vi "testLoad.vi"() -> ()   [LabVIEW 2025]
uses:
  <vilib>/userDefined/High Color/IMAQdx.ctl
  <vilib>/vision/driver/NI_Vision_Acquisition_Software.lvlib
panel:
  out "Pixel Pointer out":u64 format="%.0x"
  out "After Img 2":T1(plugin-control)
  out "Refnum out 2":T2
  out "Refnum out":T2
  out "Width":u32
  out "Height":u32
  in  "Resolution Selection 2":u16(ring)=10 items=["640x480 MJPG 30.00fps", "1280x720 MJPG 30.00fps", "1920x1080 MJPG 30.00fps", "1920x1088 MJPG 30.00fps"]
  out "video Mode names 2":string[](array[string])
  in  "Camera Selection 2":string(combo)="cam5"
  out "Camera Index list 2":string[](array[string])
  out "loadedModel":string
  out "opencvCUDA":string
  out "HostDevice":string
  in  "Sensitivity adpThScl":sgl=1.5
  out "After Img":T1(plugin-control)
  in  "stop":bool
  in  "OK Button":bool
  in  "Resolution Selection":u16(ring)=10 items=["640x480 MJPG 30.00fps", "640x480 YUY2 30.00fps", "1280x720 MJPG 30.00fps", "1280x720 YUY2 7.50fps", "1920x1080 MJPG 30.00fps", "1920x1080 YUY2 2.00fps", "2048x1536 MJPG 30.00fps", "2048x1536 YUY2 2.00fps", "2560x1440 MJPG 30.00fps", "2560x1440 YUY2 2.00fps", "3840x2160 MJPG 30.00fps", "3840x2160 YUY2 1.00fps"]
  out "video Mode names":string[](array[string])
  in  "Camera Selection":string(combo)="cam5"
  in  "confirm camera":bool
  out "Camera Index list":string[](array[string])
  out "calAdpMsg":string
  in  "Cal Img Folder Path":path=path "D:/labviewTestTCVdll/AnomalyDetection-LabVIEW/testFolder"
  out "mBBMesg":string
  out "success 2":i32
  out "successFea":u32
  out "bufferMsg":string
  out "buffer":string
  out "appended path":path
  in  "modelPath":path=path "D:/labviewTestTCVdll/AnomalyDetection-LabVIEW/models/resnet50_fp32.ts"
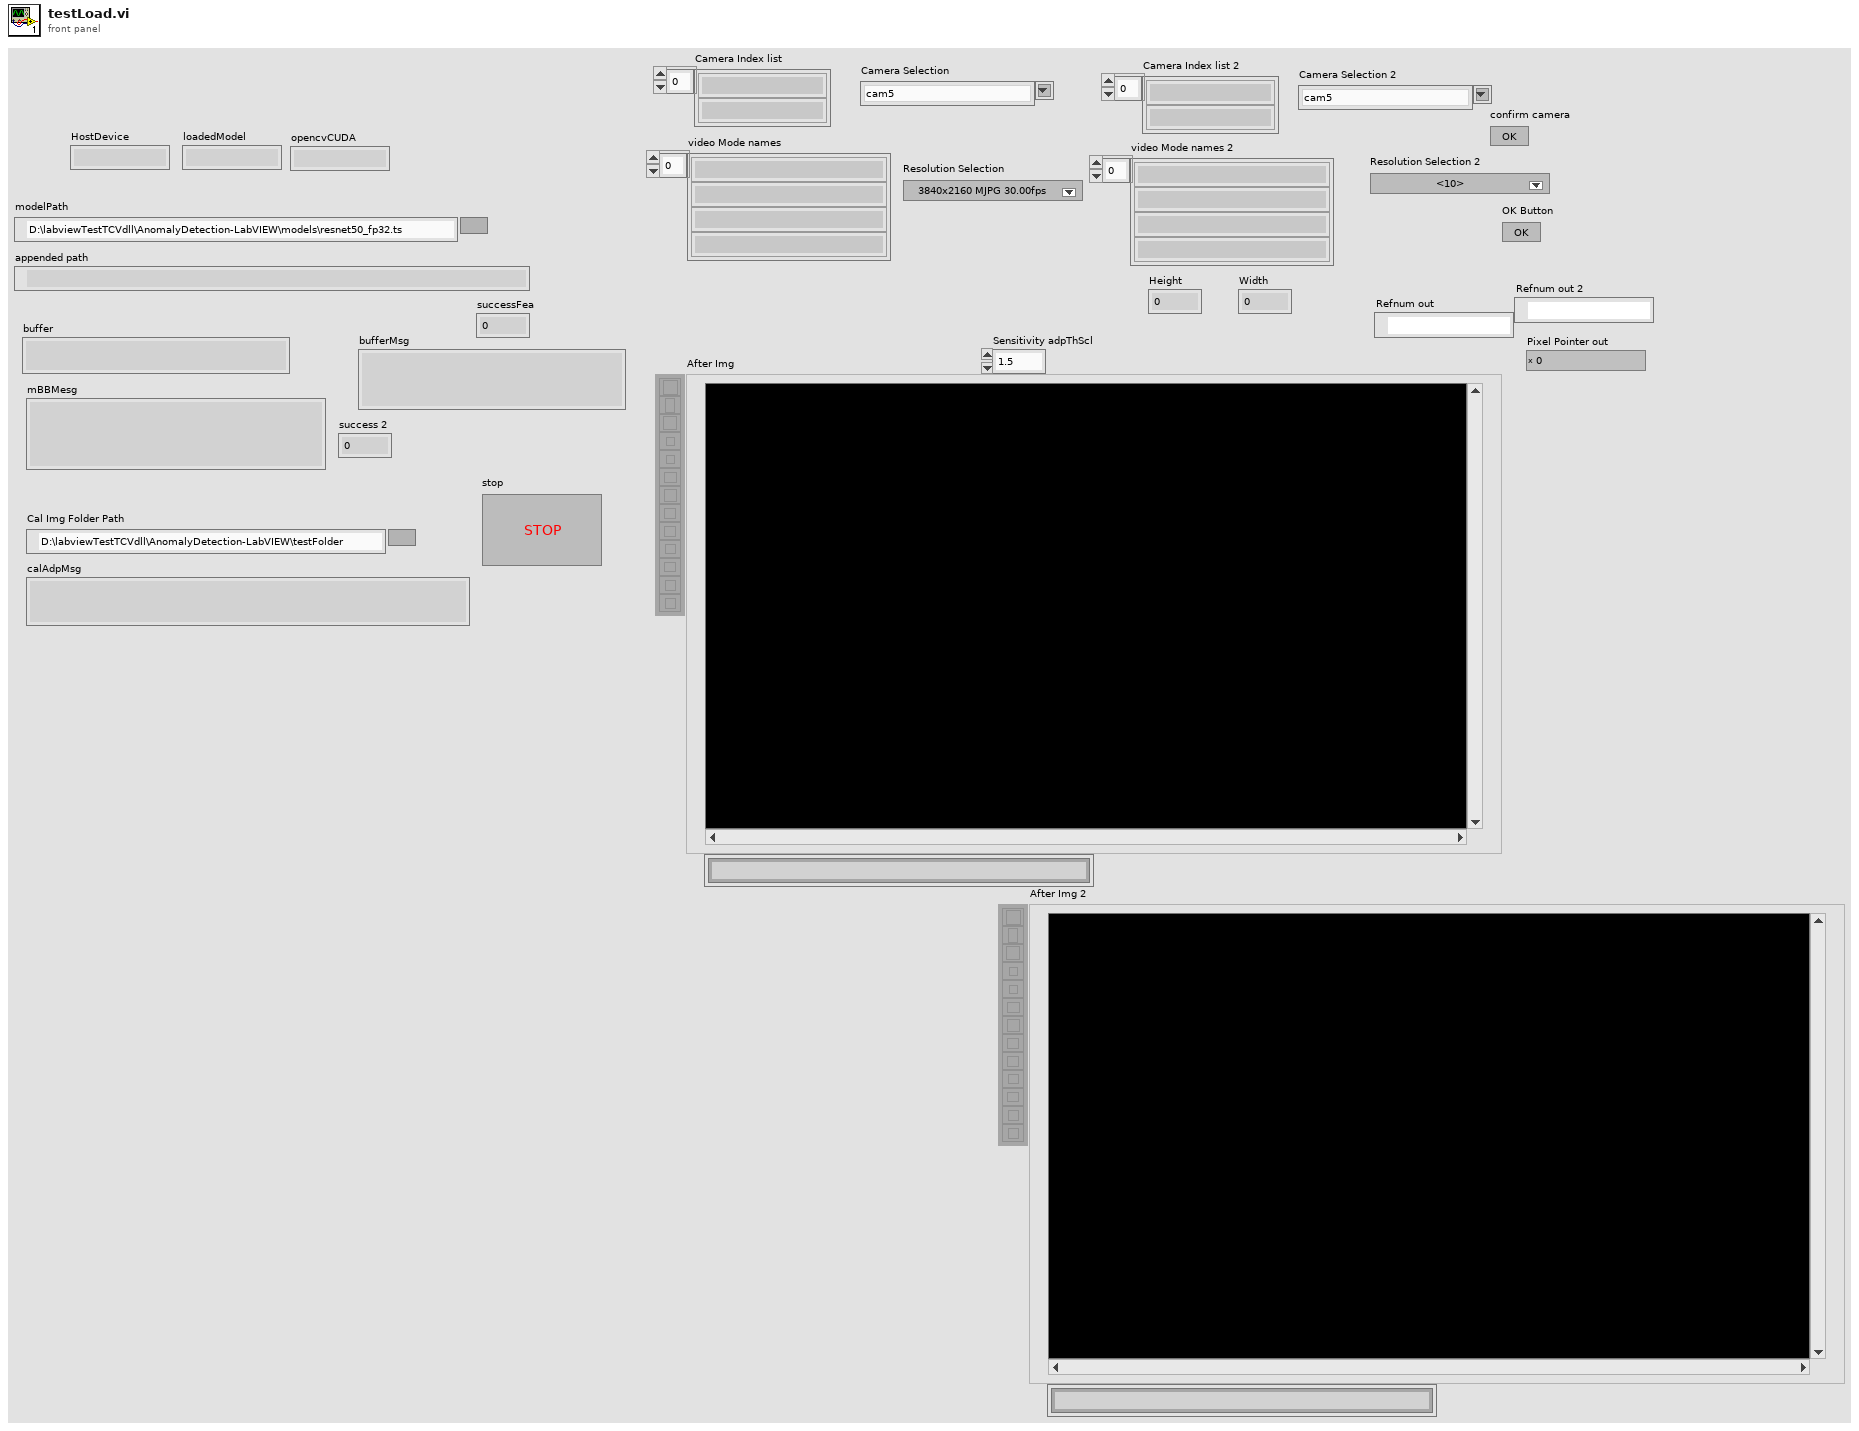
[diagram p1: front panel]
types:
  T1 = typedef "IMAQ Image.ctl" = refnum<image>
  T2 = typedef "IMAQdx.ctl" = refnum<k21>
  T3 = cluster{"Video Mode":u32, "Video Mode Name":string}[]
  T4 = enum32{"Map Pixel Pointer", "Unmap Pixel Pointer", "Get Pixels Infos"}
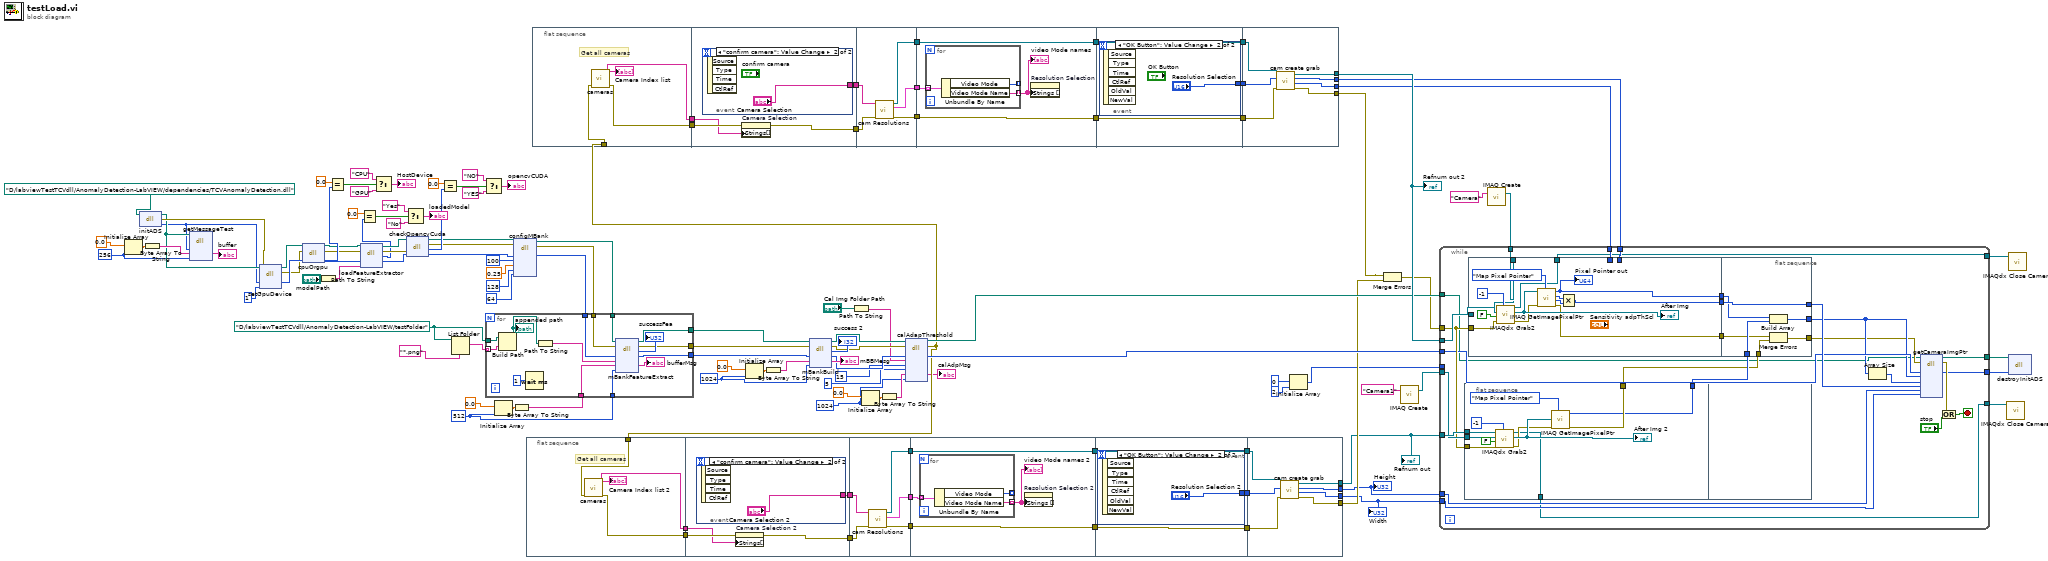
[diagram p0: block diagram]
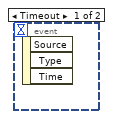
[diagram p2: hidden frame]
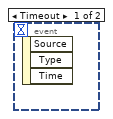
[diagram p3: hidden frame]
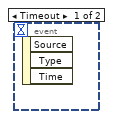
[diagram p4: hidden frame]
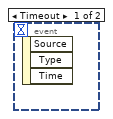
[diagram p5: hidden frame]
diagram:
  w20 = 1024 ("dimension size")
  w27 = 1024 ("dimension size")
  w33 = 512 ("dimension size")
  w5 = path "D:/labviewTestTCVdll/AnomalyDetection-LabVIEW/testFolder"
  w80 = 256 ("dimension size")
  n1 = Initialize Array(0.0 ("element"), w80) -> (w84:dbl[])
  n2 = dll-call lib="D:/labviewTestTCVdll/AnomalyDetection-LabVIEW/dependencies/TCVAnomalyDetection.dll" fn="initADS"(path in=path "D:/labviewTestTCVdll/AnomalyDetection-LabVIEW/dependencies/TCVAnomalyDetection.dll") -> (path out=w82:path, error out=w85:errorcluster, "ref"=w81:u64)  [unwired: 2 in]
  n3 = Byte Array To String(unsigned byte array=w84) -> (string=w83:string)
  n4 = dll-call lib="D:/labviewTestTCVdll/AnomalyDetection-LabVIEW/dependencies/TCVAnomalyDetection.dll" fn="getMessageTest"(path in=w82, "ref"=w81, "buffer"=w83, "size"=w80) -> ("buffer"=→"buffer":string)  [unwired: 5 in, 2 out]
  n5 = dll-call lib="D:/labviewTestTCVdll/AnomalyDetection-LabVIEW/dependencies/TCVAnomalyDetection.dll" fn="setGpuDevice"(path in=w82, error in=w85, "ref"=w81, "num"=u32 1) -> (path out=w57:path, error out=w56:errorcluster, "ref"=w58:u64)  [unwired: 3 in]
  n6 = dll-call lib="D:/labviewTestTCVdll/AnomalyDetection-LabVIEW/dependencies/TCVAnomalyDetection.dll" fn="cpuOrgpu"(path in=w57, error in=w56, "ref"=w58) -> (path out=w55:path, error out=w54:errorcluster, "ref"=w76:u64)  [unwired: 2 in]
  n7 = Path To String(path="modelPath") -> (string=w52:string)
  n8 = Equal?(x=0.0, y=w76) -> (x = y?=w75:bool)
  n9 = dll-call lib="D:/labviewTestTCVdll/AnomalyDetection-LabVIEW/dependencies/TCVAnomalyDetection.dll" fn="loadFeatureExtractor"(path in=w55, error in=w54, "ref"=w76, "path"=w52) -> (path out=w51:path, error out=w47:errorcluster, "success"=w6:i32, "ref"=w50:u64)  [unwired: 2 in]
  n10 = Equal?(x=0.0, y=w6) -> (x = y?=w8:bool)
  n11 = Select(t="CPU", s=w75, f="GPU") -> (s? t:f=→"HostDevice":string)
  n12 = dll-call lib="D:/labviewTestTCVdll/AnomalyDetection-LabVIEW/dependencies/TCVAnomalyDetection.dll" fn="checkOpencvCuda"(path in=w51, error in=w47, "ref"=w50) -> (path out=w45:path, error out=w46:errorcluster, "ocvC"=w66:i32, "ref"=w44:u64)  [unwired: 1 in]
  n13 = Select(t="Yes", s=w8, f="No") -> (s? t:f=→"loadedModel":string)
  n14 = Equal?(x=0.0, y=w66) -> (x = y?=w68:bool)
  n15 = List Folder(path=w5, pattern="*.png") -> (filenames=w48:string[])  [unwired: 2 in, 3 out]
  n16 = Select(t="NO", s=w68, f="YES") -> (s? t:f=→"opencvCUDA":string)
  n17 = Initialize Array(0.0 ("element"), w33) -> (w39:dbl[])
  n18 = Byte Array To String(unsigned byte array=w39) -> (string=w34:string)
  n19 = dll-call lib="D:/labviewTestTCVdll/AnomalyDetection-LabVIEW/dependencies/TCVAnomalyDetection.dll" fn="configMBank"(path in=w45, error in=w46, "ref"=w44, "noImages"=u32 100, "coreset"=sgl 0.25, "patchSize"=u32 128, "pathStride"=u32 64) -> (path out=w37:path, error out=w36:errorcluster, "ref"=w35:u64)  [unwired: 6 in]
  n20 = for {
    tunnel: w5 -> [w138]
    tunnel: w48 -> [w137] mode=indexing
    tunnel: w37 -> [w136]
    tunnel: w36 -> [w135]
    tunnel: w35 -> [w134]
    tunnel: w34 -> [w131]
    tunnel: w33 -> [w130]
    tunnel: [w127] -> w30
    tunnel: [w126] -> w29
    tunnel: [w125] -> w24
    n21 = Build Path(base path=w138, name or relative path=w137) -> (appended path=w133:path)
    "appended path" <- w133
    n22 = Wait (ms)(milliseconds to wait=u32 1) -> ()  [unwired: 1 out]
    n23 = Path To String(path=w133) -> (string=w132:string)
    n24 = dll-call lib="D:/labviewTestTCVdll/AnomalyDetection-LabVIEW/dependencies/TCVAnomalyDetection.dll" fn="mBankFeatureExtract"(path in=w136, error in=w135, "ref"=w134, "imagePath"=w132, "bufferMsg"=w131, "bufferSize"=w130) -> (path out=w127:path, error out=w126:errorcluster, "successFea"=→"successFea":u32, "ref"=w125:u64, "bufferMsg"=→"bufferMsg":string)  [unwired: 3 in]
  }
  n25 = flat-sequence {
    tunnel: [w141] -> w104
    tunnel: [w140] -> w103
    tunnel: w92 -> [w139]
    tunnel: w104 -> [w143]
    tunnel: w103 -> [w142]
    tunnel: [w144] -> w102
    tunnel: [w145] -> w101
    tunnel: w102 -> [w151]
    tunnel: w101 -> [w148]
    tunnel: [w149] -> w100
    tunnel: [w150] -> w99
    tunnel: [w147] -> w98
    tunnel: w100 -> [w155]
    tunnel: [w153] -> w97
    tunnel: w99 -> [w153]
    tunnel: [w152] -> w96
    tunnel: w98 -> [w152]
    tunnel: w97 -> [w161]
    tunnel: [w161] -> w95
    tunnel: w96 -> [w160]
    tunnel: [w160] -> w94
    tunnel: [w159] -> w93
    tunnel: w95 -> [w164]
    tunnel: w94 -> [w163]
    tunnel: [w167] -> w63
    tunnel: w93 -> [w169]
    tunnel: [w168] -> w86
    tunnel: [w166] -> w88
    tunnel: [w165] -> w64
    frame #0 {
      # "Get all cameras"
      n26 = call "cameras.vi"("error in"=w139) -> ("error out"=w141:errorcluster, "Array"=w140:string[])  [unwired: 9 in]
      "Camera Index list 2" <- w140
    }
    frame #1 {
      n27 = event shown="[1] \"confirm camera\": Value Change" {
        selector: _ -> [_ _]
        dyn-events: _ -> [_ _]
        timeout: _ -> [_ _]
        tunnel: [_ "Camera Selection 2"] -> w144
        event Timeout {
          n28 = event-data() -> ()  [unwired: 1 in, 3 out]
        }
        event "confirm camera": Value Change {
          n29 = event-data() -> ()  [unwired: 1 in, 4 out]
        }
      }
      n30 = property on="Camera Selection 2" class="CmbBox"(error in=w143, "Strings[]"=w142) -> (error out=w145:errorcluster)  [unwired: 1 in, 1 out]
    }
    frame #2 {
      n31 = call "cam Resolutions.vi"("error in (no error)"=w148, "Camera Selection"=w151) -> ("error out"=w147:errorcluster, "Video Modes"=w149:T3, "Refnum out"=w150:T2)  [unwired: 7 in]
    }
    frame #3 {
      n32 = for {
        tunnel: w155 -> [w158] mode=indexing
        tunnel: [w157] -> _ mode=indexing
        tunnel: [w156] -> w154 mode=indexing
        n33 = Unbundle By Name(w158) -> ("Video Mode"=w157:u32, "Video Mode Name"=w156:string)
      }
      "video Mode names 2" <- w154
      n34 = property on="Resolution Selection 2" class="Ring (strict)"("Strings []"=w154) -> ()  [unwired: 2 in, 2 out]
    }
    frame #4 {
      n35 = event shown="[1] \"OK Button\": Value Change" {
        selector: _ -> [_ _]
        dyn-events: _ -> [_ _]
        timeout: _ -> [_ _]
        tunnel: [_ "Resolution Selection 2"] -> w159
        event Timeout {
          n36 = event-data() -> ()  [unwired: 1 in, 3 out]
        }
        event "OK Button": Value Change {
          n37 = event-data() -> ()  [unwired: 1 in, 6 out]
        }
      }
    }
    frame #5 {
      n38 = call "cam create grab.vi"("error in (no error)"=w163, "Resolution Selection"=w169, "Refnum in"=w164) -> ("error out"=w166:errorcluster, "Width"=w165:u32, "Height"=w167:u32, "Refnum out"=w168:T2)  [unwired: 5 in]
    }
  }
  n39 = flat-sequence {
    tunnel: [w172] -> w123
    tunnel: [w171] -> w122
    tunnel: w92 -> [w170]
    tunnel: w123 -> [w174]
    tunnel: w122 -> [w173]
    tunnel: [w175] -> w121
    tunnel: [w176] -> w120
    tunnel: w121 -> [w182]
    tunnel: w120 -> [w179]
    tunnel: [w180] -> w119
    tunnel: [w181] -> w118
    tunnel: [w178] -> w117
    tunnel: w119 -> [w186]
    tunnel: [w184] -> w116
    tunnel: w118 -> [w184]
    tunnel: [w183] -> w115
    tunnel: w117 -> [w183]
    tunnel: w116 -> [w192]
    tunnel: [w192] -> w114
    tunnel: w115 -> [w191]
    tunnel: [w191] -> w113
    tunnel: [w190] -> w112
    tunnel: w114 -> [w195]
    tunnel: w113 -> [w194]
    tunnel: [w198] -> w108
    tunnel: w112 -> [w200]
    tunnel: [w199] -> w111
    tunnel: [w197] -> w89
    tunnel: [w196] -> w109
    frame #0 {
      # "Get all cameras"
      n40 = call "cameras.vi"("error in"=w170) -> ("error out"=w172:errorcluster, "Array"=w171:string[])  [unwired: 9 in]
      "Camera Index list" <- w171
    }
    frame #1 {
      n41 = event shown="[1] \"confirm camera\": Value Change" {
        selector: _ -> [_ _]
        dyn-events: _ -> [_ _]
        timeout: _ -> [_ _]
        tunnel: [_ "Camera Selection"] -> w175
        event Timeout {
          n42 = event-data() -> ()  [unwired: 1 in, 3 out]
        }
        event "confirm camera": Value Change {
          n43 = event-data() -> ()  [unwired: 1 in, 4 out]
        }
      }
      n44 = property on="Camera Selection" class="CmbBox"(error in=w174, "Strings[]"=w173) -> (error out=w176:errorcluster)  [unwired: 1 in, 1 out]
    }
    frame #2 {
      n45 = call "cam Resolutions.vi"("error in (no error)"=w179, "Camera Selection"=w182) -> ("error out"=w178:errorcluster, "Video Modes"=w180:T3, "Refnum out"=w181:T2)  [unwired: 7 in]
    }
    frame #3 {
      n46 = for {
        tunnel: w186 -> [w189] mode=indexing
        tunnel: [w188] -> _ mode=indexing
        tunnel: [w187] -> w185 mode=indexing
        n47 = Unbundle By Name(w189) -> ("Video Mode"=w188:u32, "Video Mode Name"=w187:string)
      }
      "video Mode names" <- w185
      n48 = property on="Resolution Selection" class="Ring (strict)"("Strings []"=w185) -> ()  [unwired: 2 in, 2 out]
    }
    frame #4 {
      n49 = event shown="[1] \"OK Button\": Value Change" {
        selector: _ -> [_ _]
        dyn-events: _ -> [_ _]
        timeout: _ -> [_ _]
        tunnel: [_ "Resolution Selection"] -> w190
        event Timeout {
          n50 = event-data() -> ()  [unwired: 1 in, 3 out]
        }
        event "OK Button": Value Change {
          n51 = event-data() -> ()  [unwired: 1 in, 6 out]
        }
      }
    }
    frame #5 {
      n52 = call "cam create grab.vi"("error in (no error)"=w194, "Resolution Selection"=w200, "Refnum in"=w195) -> ("error out"=w197:errorcluster, "Width"=w196:u32, "Height"=w198:u32, "Refnum out"=w199:T2)  [unwired: 5 in]
    }
  }
  n53 = Initialize Array(0.0 ("element"), w27) -> (w31:dbl[])
  n54 = Byte Array To String(unsigned byte array=w31) -> (string=w28:string)
  n55 = dll-call lib="D:/labviewTestTCVdll/AnomalyDetection-LabVIEW/dependencies/TCVAnomalyDetection.dll" fn="mBankBuild"(path in=w30, error in=w29, "ref"=w24, "mBBMesg"=w28, "bufferSize"=w27) -> (path out=w19:path, error out=w18:errorcluster, "success"=→"success 2":i32, "ref"=w17:u64, "mBBMesg"=→"mBBMesg":string)  [unwired: 2 in]
  n56 = Path To String(path="Cal Img Folder Path") -> (string=w13:string)
  n57 = Initialize Array(0.0 ("element"), w20) -> (w23:dbl[])
  n58 = Byte Array To String(unsigned byte array=w23) -> (string=w21:string)
  n59 = dll-call lib="D:/labviewTestTCVdll/AnomalyDetection-LabVIEW/dependencies/TCVAnomalyDetection.dll" fn="calAdapThreshold"(path in=w19, error in=w18, "ref"=w17, "calImgfolderPath"=w13, "noCalImg"=u32 15, "NumNearsesNei"=u32 5, "calAdpMsg"=w21, "bufferSize"=w20) -> (path out=w110:path, error out=w92:errorcluster, "ref"=w107:u64, "calAdpMsg"=→"calAdpMsg":string)  [unwired: 6 in]
  n60 = Initialize Array(u64 0 ("element"), 2 ("dimension size")) -> (w60:u64[])
  n61 = Merge Errors(w89, w88) -> (w87:errorcluster)
  n62 = call "IMAQ Create"("Image Name"="Camera1") -> ("New Image"=w105:T1)  [unwired: 4 in, 1 out]
  n63 = call "IMAQ Create"("Image Name"="Camera") -> ("New Image"=w90:T1)  [unwired: 4 in, 1 out]
  n64 = while {
    tunnel: w90 -> [w227]
    tunnel: w111 -> [w226]
    tunnel: w87 -> [w221]
    tunnel: w110 -> [w205]
    tunnel: w109 -> [w224]
    tunnel: w108 -> [w225]
    tunnel: w107 -> [w214]
    tunnel: w105 -> [w222]
    tunnel: w86 -> [w223]
    tunnel: w64 -> [w219]
    tunnel: w63 -> [w220]
    tunnel: w60 -> [_]
    tunnel: [w204] -> w4
    tunnel: [w203] -> w3
    tunnel: [w202] -> w2
    tunnel: [w201] -> w1
    stop <- w213 stop-if-true
    n65 = flat-sequence {
      tunnel: w223 -> [w238]
      tunnel: w222 -> [w237]
      tunnel: w221 -> [w234]
      tunnel: [w230] -> w208
      tunnel: [w229] -> w209
      tunnel: [w228] -> w204
      frame #0 {
        n66 = call <vilib>:"IMAQdx Grab2.vi"("Timeout (ms)"=-1, "error in"=w234, "Wait for Next Buffer? (Yes)"=FALSE, "Image In"=w237, "Session In"=w238) -> ("error out"=w231:errorcluster, "Image Out"=w232:T1, "Session Out"=w228:T2)  [unwired: 3 in, 1 out]
        "After Img 2" <- w232
        n67 = call "IMAQ GetImagePixelPtr"("Function"=T4."Map Pixel Pointer", "error in (no error)"=w231, "Image"=w232) -> ("error out"=w230:errorcluster, "Pixel Pointer out"=w229:u64)  [unwired: 3 in, 4 out]
      }
      frame #1 {
      }
    }
    n68 = flat-sequence {
      tunnel: w221 -> [w245]
      tunnel: w227 -> [w250]
      tunnel: w226 -> [w249]
      tunnel: w225 -> [_]
      tunnel: w224 -> [_]
      tunnel: [w243] -> w217
      tunnel: [w242] -> w216
      tunnel: [w240] -> w206
      tunnel: [w239] -> w203
      tunnel: [w259] -> w218
      tunnel: w217 -> [w259]
      tunnel: w216 -> [w258]
      tunnel: [w257] -> w210
      tunnel: w209 -> [w256]
      tunnel: w208 -> [w255]
      tunnel: [w254] -> w207
      tunnel: w206 -> [w253]
      frame #0 {
        n69 = call <vilib>:"IMAQdx Grab2.vi"("Timeout (ms)"=-1, "error in"=w245, "Wait for Next Buffer? (Yes)"=FALSE, "Image In"=w250, "Session In"=w249) -> ("error out"=w241:errorcluster, "Image Out"=w244:T1, "Session Out"=w239:T2)  [unwired: 3 in, 1 out]
        "After Img" <- w244
        n70 = call "IMAQ GetImagePixelPtr"("Function"=T4."Map Pixel Pointer", "error in (no error)"=w241, "Image"=w244) -> ("error out"=w240:errorcluster, "Pixel Size (Bytes)"=w247:i32, "LineWidth(Pixels)"=w248:i32, "Pixel Pointer out"=w242:u64)  [unwired: 3 in, 2 out]
        "Pixel Pointer out" <- w242
        n71 = Multiply(x=w248, y=w247) -> (x*y=w243:i32)
      }
      frame #1 {
        n72 = Build Array(w258, w256) -> (w257:u64[])
        n73 = Merge Errors(w253, w255) -> (w254:errorcluster)
      }
    }
    n74 = Array Size(array=w210) -> (size(s)=w215:i32)
    n75 = dll-call lib="D:/labviewTestTCVdll/AnomalyDetection-LabVIEW/dependencies/TCVAnomalyDetection.dll" fn="getCameraImgPtr"(path in=w205, error in=w207, "ref"=w214, "imgPtrs"=w210, "noCamers"=w215, "lw"=w218, "h"=w220, "w"=w219) -> (path out=w202:path, error out=w211:errorcluster, "ref"=w201:u64)  [unwired: 7 in]
    n76 = Or(x=w211, y="stop") -> (x .or. y?=w213:bool)
  }
  n77 = call <vilib>:"IMAQdx Close Camera.vi"("Session In"=w4) -> ()  [unwired: 10 in, 1 out]
  n78 = call <vilib>:"IMAQdx Close Camera.vi"("Session In"=w3) -> ()  [unwired: 10 in, 1 out]
  n79 = dll-call lib="D:/labviewTestTCVdll/AnomalyDetection-LabVIEW/dependencies/TCVAnomalyDetection.dll" fn="destroyInitADS"(path in=w2, "ref"=w1) -> ()  [unwired: 4 in, 2 out]
  "Height" <- w63
  "Width" <- w64
  "Refnum out" <- w86
  "Refnum out 2" <- w111
